vi "gyro_data.vi"() -> ()   [LabVIEW 2014]
uses:
  <vilib>/Platform/TimedLoop/XDataNode/timing_clust.ctl
  <vilib>/Platform/TimedLoop/XDataNode/nitl_modes.ctl
  <vilib>/Platform/TimedLoop/XDataNode/wakeup.ctl
  <vilib>/Analysis/3filter.llb/Filter Passband Type.ctl
  <vilib>/myRIO/Instrument Drivers/Onboard IO/AI/vis/Read.vi
  <vilib>/myRIO/Instrument Drivers/Onboard IO/AI/vis/Smart Open.vi
  <vilib>/Utility/error.llb/Error Cluster From Error Code.vi
  <vilib>/myRIO/Common/Instrument Driver Framework/myRIO v1.0/AI/vis/myRIO v1.0 Read AI.vi
  <vilib>/platform/TimedLoop/XDataNode/XDataNode.xnode
  <vilib>/Platform/TimedLoop/XDataNode/XDNodeRunTimeDep.lvlib
  <vilib>/ptbypt/NI_PtbyPt.lvlib
  <vilib>/Analysis/NI_AALBase.lvlib
panel:
  out "Angluar Rate-Average":dbl
  out "Angluar Rate":dbl
  out "Angle Rate-Average":dbl(graph)
  in  "initialize_org":bool
  out "Angluar Rate 2":dbl(graph)
  out "Angluar Rate_Butterworth":dbl(graph)
  out "Angle_Butterworth":dbl(graph)
  in  "initialize_Butterworth":bool
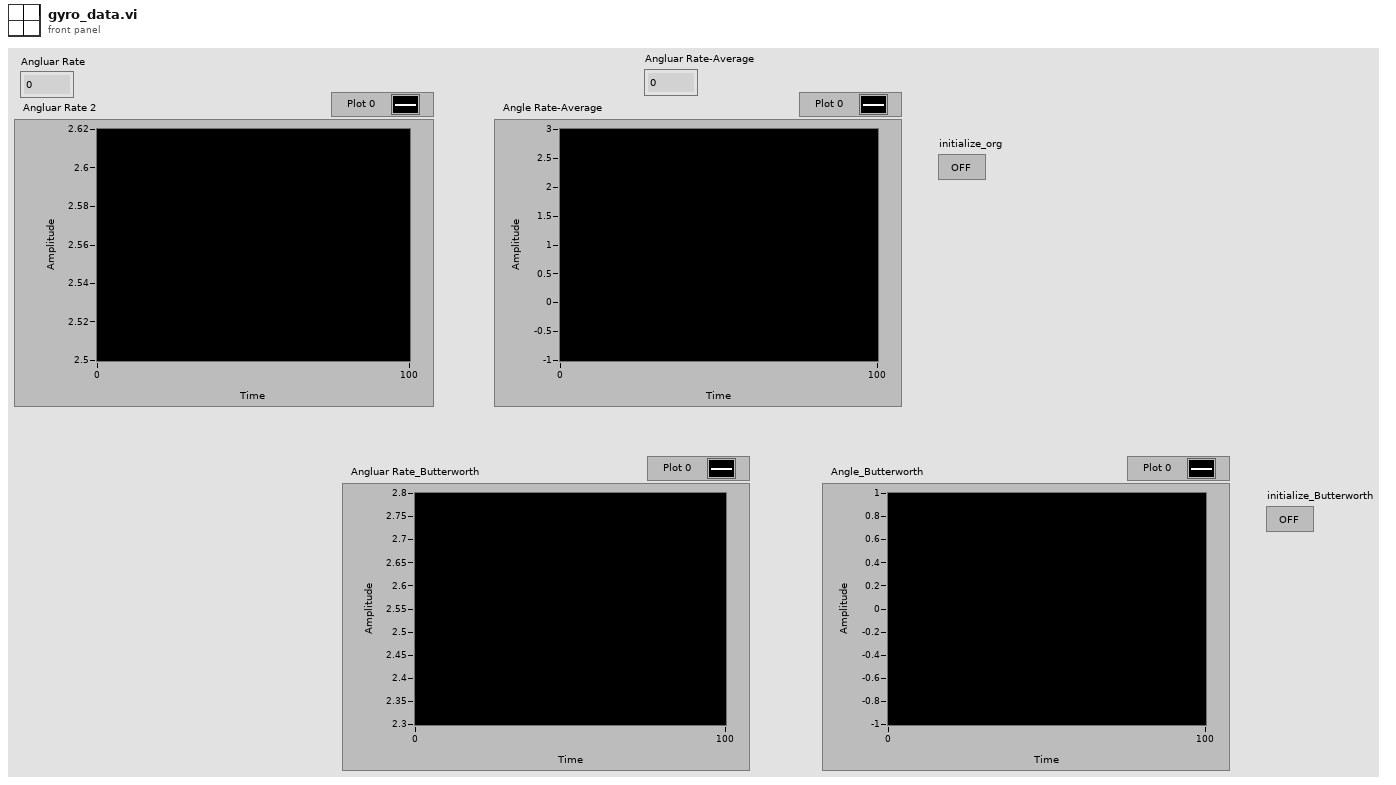
[diagram p1: front panel]
types:
  T1 = typedef "XDNodeRunTimeDep.lvlib/timing_clust.ctl" = cluster{"Expected End [f-1]":u64, "Actual End [f-1]":u64, "Finished Late? [f-1]":bool, "Expected End [i-1]":u64, "Actual End [i-1]":u64, "Finished Late? [i-1]":bool, "Expected Start [i]":u64, "Actual Start [i]":u64, "Expected Start [f]":u64, "Actual Start [f]":u64, "Source Name":string, "Structure Name":string, "Period":i64, "Deadline":i64, "Offset":i64, "Start":i64, "Priority":i32, "Timeout":i32, "Mode":T2, "Wakeup Reason":T3, "Error":errorcluster, "Source Type":string, "Secondary Source Type":string, "Global End Time":u64, "Global Start Time":u64, "Frame Duration":u64, "Iteration Duration":u64, "Assigned CPU":i32, "I/O Scan Engine Mode":u32}
  T2 = typedef "XDNodeRunTimeDep.lvlib/nitl_modes.ctl" = enum32{"No Change", "Process missed periods, maintain original phase", "Discard missed periods, maintain original phase", "Process missed periods, ignore original phase", "Discard missed periods, ignore original phase"}
  T3 = typedef "XDNodeRunTimeDep.lvlib/wakeup.ctl" = enum32{"Normal", "Aborted", "Asynchronous wakeup", "Timing source error", "Timed loop error", "Timeout"}
  T4 = typedef "NI_AALBase.lvlib/Filter Passband Type.ctl" = enum32{"Lowpass", "Highpass", "Bandpass", "Bandstop"}
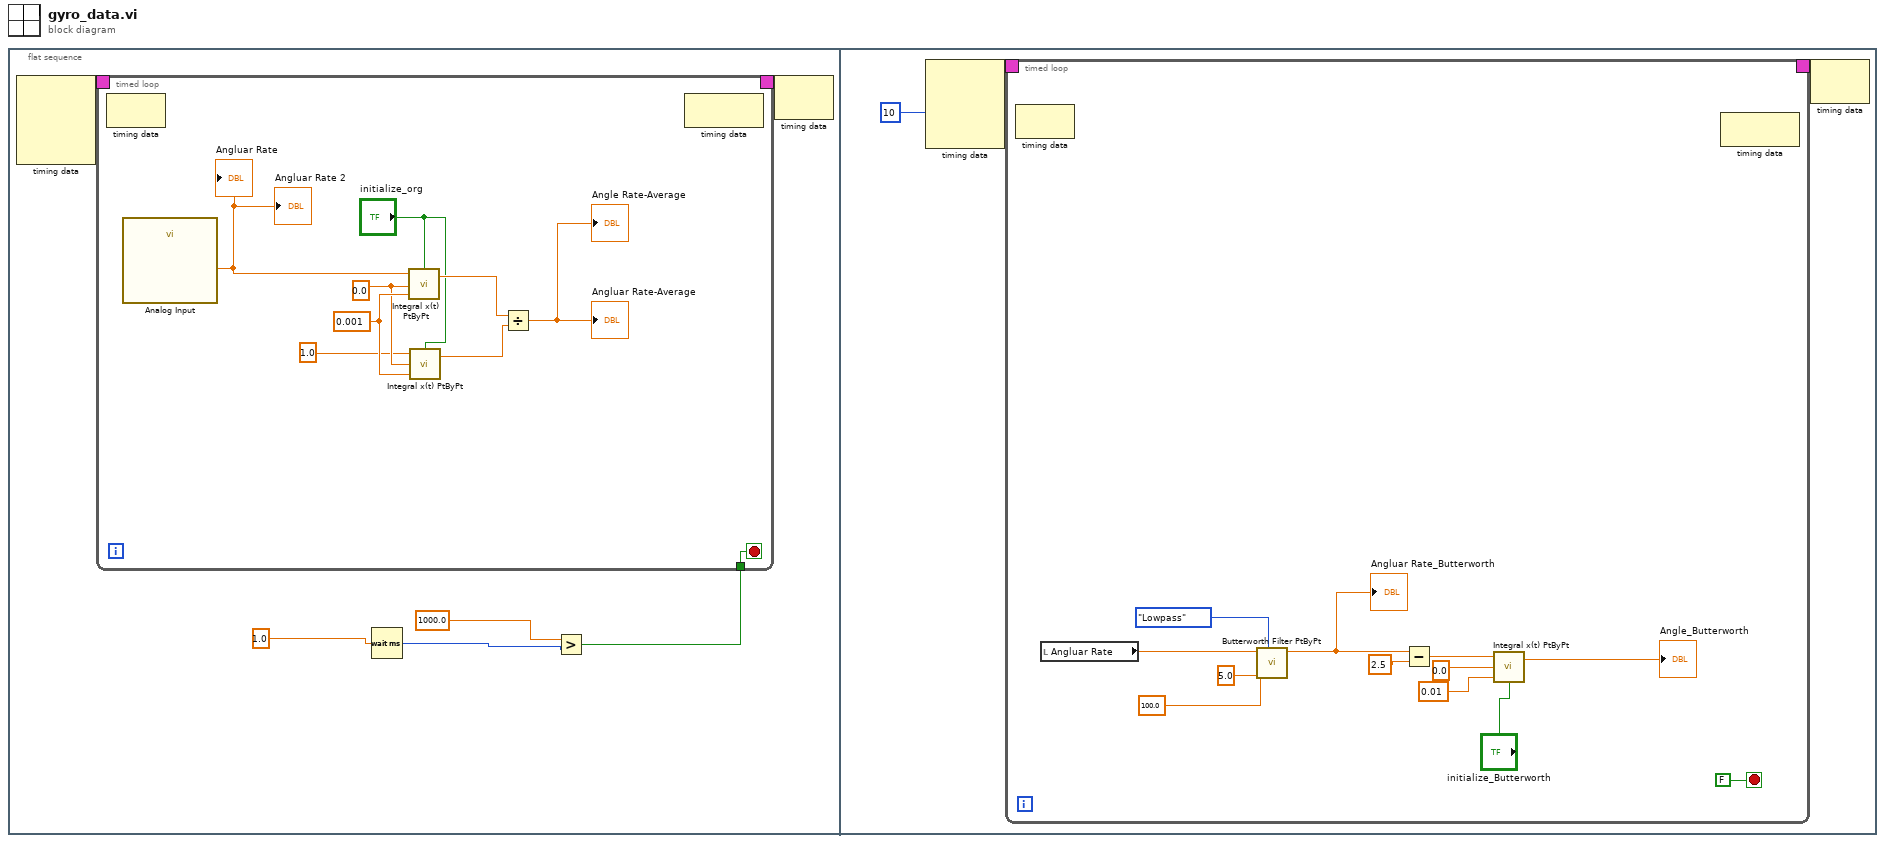
[diagram p0: block diagram]
diagram:
  n1 = flat-sequence {
    frame #0 {
      n2 = node-c288() -> (w6:T1)  [unwired: 4 in]
      n3 = Wait (ms)(milliseconds to wait=1.0 ("dt")) -> (millisecond timer value=w3:u32)
      n4 = Greater?(x=1000.0 ("dt"), y=w3) -> (0:w1:bool)
      n5 = timed-loop {
        timing: w6 -> [_]
        timing-out: [_] -> w5
        tunnel: w1 -> [w7]
        stop <- w7 stop-if-true
        w14 = 0.001 ("dt")
        w13 = 0.0 ("initial condition")
        n6 = node-c288() -> ()  [unwired: 1 in, 1 out]
        n7 = call "Analog Input"() -> ("B/AI0 (Pin 3)"=w15:dbl)  [unwired: 26 in, 1 out]
        "Angluar Rate 2" <- w15
        "Angluar Rate" <- w15
        n8 = call <vilib>:"Integral x(t) PtByPt.vi"("initialize"="initialize_org", "dt"=w14, "initial condition"=w13, "x"=w15) -> ("integral x(t)"=w11:dbl)  [unwired: 1 out]
        n9 = call <vilib>:"Integral x(t) PtByPt.vi"("initialize"="initialize_org", "dt"=w14, "initial condition"=w13, "x"=1.0 ("dt")) -> ("integral x(t)"=w10:dbl)  [unwired: 1 out]
        n10 = Divide(x=w11, y=w10) -> (x/y=→"Angle Rate-Average" →"Angluar Rate-Average":dbl)
        n11 = node-c288() -> ()  [unwired: 1 in, 1 out]
      }
      n12 = node-c288(w5) -> ()  [unwired: 1 out]
    }
    frame #1 {
      n13 = node-c288(i64 10 ("Period")) -> (w22:T1)  [unwired: 3 in]
      n14 = timed-loop {
        timing: w22 -> [_]
        timing-out: [_] -> w21
        stop <- FALSE stop-if-true
        n15 = node-c288() -> ()  [unwired: 1 in, 1 out]
        n16 = local read "Angluar Rate"() -> (w23:dbl)
        n17 = call <vilib>:"Butterworth Filter PtByPt.vi"("filter type"=Filter_Passband_Type."Lowpass", "low cutoff freq: fl"=5.0, "sampling freq: fs"=100.0, "x"=w23) -> ("Filtered x"=w26:dbl)  [unwired: 5 in, 1 out]
        "Angluar Rate_Butterworth" <- w26
        n18 = Subtract(x=w26, y=2.5) -> (x-y=w27:dbl)
        n19 = call <vilib>:"Integral x(t) PtByPt.vi"("initialize"="initialize_Butterworth", "dt"=0.01, "initial condition"=0.0, "x"=w27) -> ("integral x(t)"=→"Angle_Butterworth":dbl)  [unwired: 1 out]
        n20 = node-c288() -> ()  [unwired: 1 in, 1 out]
      }
      n21 = node-c288(w21) -> ()  [unwired: 1 out]
    }
  }
